vi "niUSRP Tx Continuous Lab.vi"() -> ()   [LabVIEW 2014]
uses:
  <vilib>/measure/maspectr.llb/FFT Power Spectrum and PSD for 1 Chan (CDB).vi
  <instrlib>/niUSRP/niUSRP Write Tx Data (CDB).vi
  <vilib>/measure/NI_MAPro.lvlib
  <vilib>/measure/NI_MABase.lvlib
panel:
  in  "offset 2":dbl format="%0.2p"
  in  "offset":dbl format="%0.2p"
  in  "Stop Button":bool
  out "Frequency Plot":cluster{"f0":dbl, "df":dbl, "magnitude":dbl[]}(graph)
  out "IQ Plot":waveform(dbl)[](graph)
  in  "device name":refnum<k15>="192.168.10.2"
  out "Error Out":errorcluster
  in  "active antenna":string="TX/RX"
  in  "tone frequency":dbl=10000.0 format="%#_6p"
  in  "waveform size":dbl=10000.0
  out "Gain [dB] (actual)":dbl format="%#.6p"
  out "Carrier Frequency \n[Hz] (actual)":dbl=2450000000.0 format="%#.6p"
  out "IQ Sampling\nRate [s/sec] (actual)":dbl=10000000.0 format="%#.6p"
  in  "Gain [dB]":dbl format="%#.6p"
  in  "Carrier\nFrequency [Hz]":dbl=915000000.0 format="%#.6p"
  in  "IQ Sampling\nRate [s/sec]":dbl=10000000.0 format="%#.6p"
  # "IQ Transmitter"
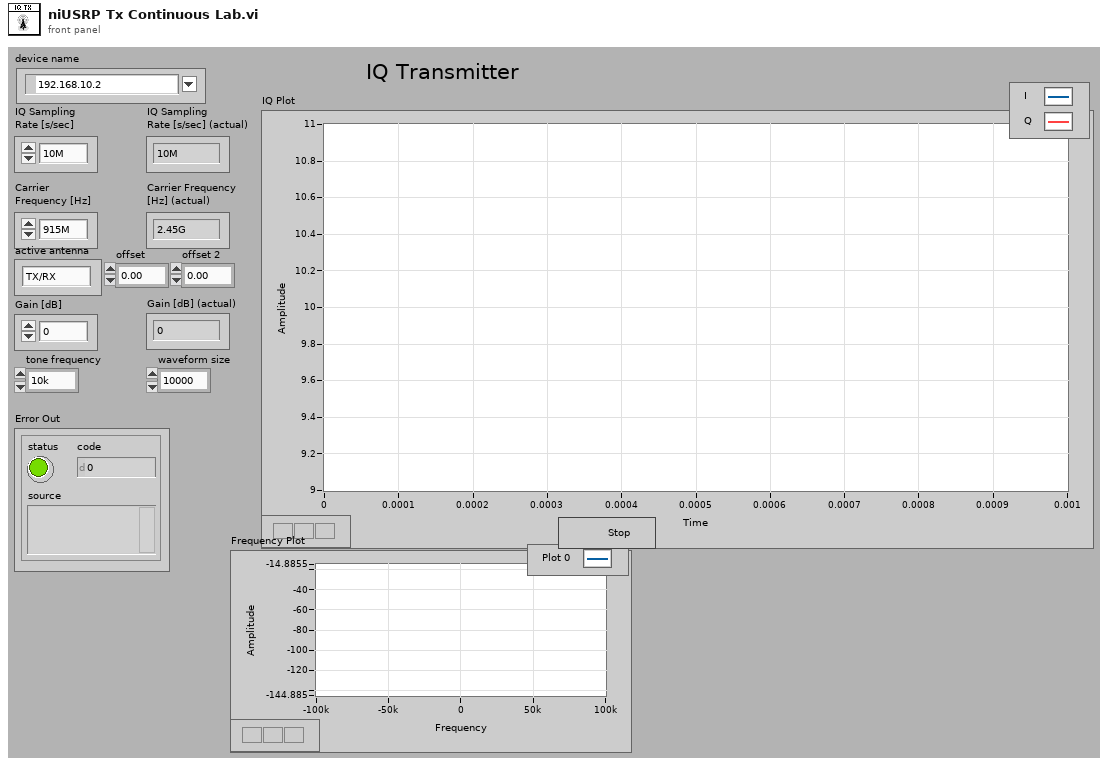
[diagram p1: front panel]
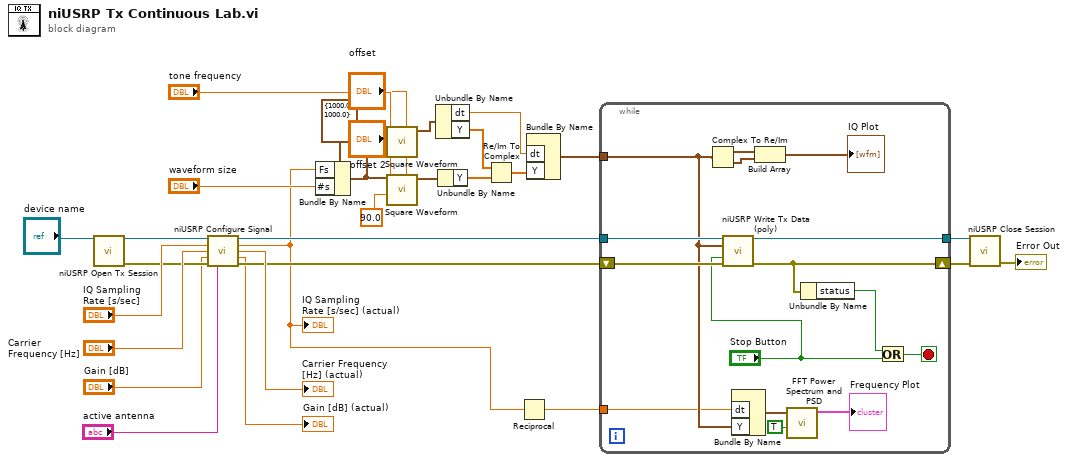
[diagram p0: block diagram]
diagram:
  n1 = call <instrlib>:"niUSRP Open Tx Session.vi"("device names"="device name") -> ("session handle out"=w30:refnum<k15>, "error out"=w27:errorcluster)  [unwired: 13 in]
  n2 = call <instrlib>:"niUSRP Configure Signal.vi"("session handle"=w30, "IQ rate"="IQ Sampling\nRate [s/sec]", "carrier frequency"="Carrier\nFrequency [Hz]", "gain"="Gain [dB]", "error in (no error)"=w27, "active antenna"="active antenna") -> ("session handle out"=w25:refnum<k15>, "coerced IQ rate"=w7:dbl, "coerced carrier frequency"=→"Carrier Frequency \n[Hz] (actual)":dbl, "coerced gain"=→"Gain [dB] (actual)":dbl, "error out"=w24:errorcluster)  [unwired: 5 in]
  "IQ Sampling\nRate [s/sec] (actual)" <- w7
  n3 = Bundle By Name(cluster=cluster{"Fs":dbl, "#s":dbl} {"Fs"=1000.0, "#s"=1000.0} ("sampling info"), "Fs"=w7, "#s"="waveform size") -> (w19:cluster{"Fs":dbl, "#s":dbl})
  n4 = call <vilib>:"Square Waveform.vi"("offset"="offset", "sampling info"=w19, "frequency"="tone frequency") -> ("signal out"=w15:waveform(dbl))  [unwired: 7 in, 1 out]
  n5 = call <vilib>:"Square Waveform.vi"("offset"="offset 2", "sampling info"=w19, "phase"=90.0, "frequency"="tone frequency") -> ("signal out"=w16:waveform(dbl))  [unwired: 6 in, 1 out]
  n6 = Unbundle By Name(w15) -> ("dt"=w5:dbl, "Y"=w14:dbl[])
  n7 = Unbundle By Name(w16) -> ("Y"=w13:dbl[])
  n8 = Re/Im To Complex(1:w13, 2:w14) -> (0:w4:cdb[])
  n9 = Reciprocal(x=w7) -> (1/x=w8:dbl)
  n10 = Bundle By Name("dt"=w5, "Y"=w4) -> (w3:waveform(cdb))  [unwired: 1 in]
  n11 = while {
    tunnel: w25 -> [w43]
    tunnel: [w41] -> w23
    shift-right: [w40] -> w22
    shift-left: w24 -> [w42]
    tunnel: w3 -> [w36]
    tunnel: w8 -> [w35]
    stop <- w45 stop-if-true
    n12 = Complex To Re/Im(x + iy=w36) -> (x=w37:waveform(dbl), y=w38:waveform(dbl))
    n13 = call-poly <instrlib>:"niUSRP Write Tx Data (poly).vi"("session handle"=w43, "data"=w36, "end of data?"="Stop Button", "error in (no error)"=w42) -> ("session handle out"=w41:refnum<k15>, "error out"=w40:errorcluster)  [unwired: 10 in]
    n14 = Bundle By Name("dt"=w35, "Y"=w36) -> (w39:waveform(cdb))  [unwired: 1 in]
    n15 = Build Array(w37, w38) -> (→"IQ Plot":waveform(dbl)[])
    n16 = call-poly <vilib>:"FFT Power Spectrum and PSD.vi"("dB On (F)"=TRUE, "time signal"=w39) -> ("Power Spectrum / PSD"=→"Frequency Plot":cluster{"f0":dbl, "df":dbl, "magnitude":dbl[]})  [unwired: 6 in, 3 out]
    n17 = Unbundle By Name(w40) -> ("status"=w44:bool)
    n18 = Or(x=w44, y="Stop Button") -> (x .or. y?=w45:bool)
  }
  n19 = call <instrlib>:"niUSRP Close Session.vi"("session handle"=w23, "error in (no error)"=w22) -> ("error out"=→"Error Out":errorcluster)  [unwired: 13 in]
